vi "Main.vi"() -> ()   [LabVIEW 2018]
panel:
  in  "For Debugging:":bool
  out "State":dbl
  in  "Tab Control":T1(tab)
  out "Mass Flow":dbl(knob) scale=0.0..10.0
  out "Transducer Part":dbl(slide) scale=0.0..10.0
  out "Transducer Source":dbl(slide) scale=0.0..10.0
  out "Thermocouple Part":dbl(slide) scale=0.0..600.0
  out "Thermocouple Source":dbl(slide) scale=0.0..600.0
  in  "Select Default Process":bool
  out "Waveform Graph":waveform(dbl)(graph)
  out "Status Feed":string
  in  "Standard Processes":string(combo)
  out "Valid Process":bool
  in  "ABORT":bool
  in  "Start":bool
  out "Progression":u8(slide) scale=0.0..100.0
  out "DANGER":bool
  in  "Save File(s) Location":path
  in  "Emergency Contact (Carrier)":enum16{"T-Mobile", "AT&T", "Verizon", "Sprint"}(ring)
  in  "Emergency Contact (phone number)":string
  in  "Name of Experiment":string="LabVIEW Error"
  in  "Centigrade / Fahrenheit":bool
  in  "Set Schedules":bool
  in  "Clear Mass Flow Schedule":bool
  in  "Clear Pressure Schedule":bool
  in  "Clear Temp Schedule":bool
  in  "Mass Flow Process Schedule":T2(array[cluster])
  in  "Pressure Process Schedule":T2(array[cluster])
  in  "Temperature Process Schedule":T3(array[cluster])
  in  "Max Rate Temperature 3":dbl
  in  "Min Temperature 3":dbl
  in  "Max Temperature 3":dbl
  in  "Max Rate Temperature 2":dbl
  in  "Min Temperature 2":dbl
  in  "Max Temperature 2":dbl
  in  "Max Rate Temperature":dbl=10.0
  in  "Min Temperature":dbl=25.0
  in  "Max Temperature":dbl=600.0
  out "Input Validated":bool
  out "Initialized":bool
  # "BLUE M SINGLEZONE FURNACE: SKELETON CODE"
  # "Temperature Readings"
  # "Pressure Readings"
  # "Mass Flow Readings"
  # "Temperature Settings"
  # "Mass Flow Settings"
  # "These represent the max allowable settings for the process. It is recommended that temperature limits should be set well within the safety limits of the equipment. Please allow generous safety margins!"
  # "These represent the max allowable settings for the process. It is recommended that temperature limits should be set well within the safety limits of the equipment. Please allow generous safety margins!"
  # "Pressure Settings"
  # "These represent the max allowable settings for the process. It is recommended that temperature limits should be set well within the safety limits of the equipment. Please allow generous safety margins!"
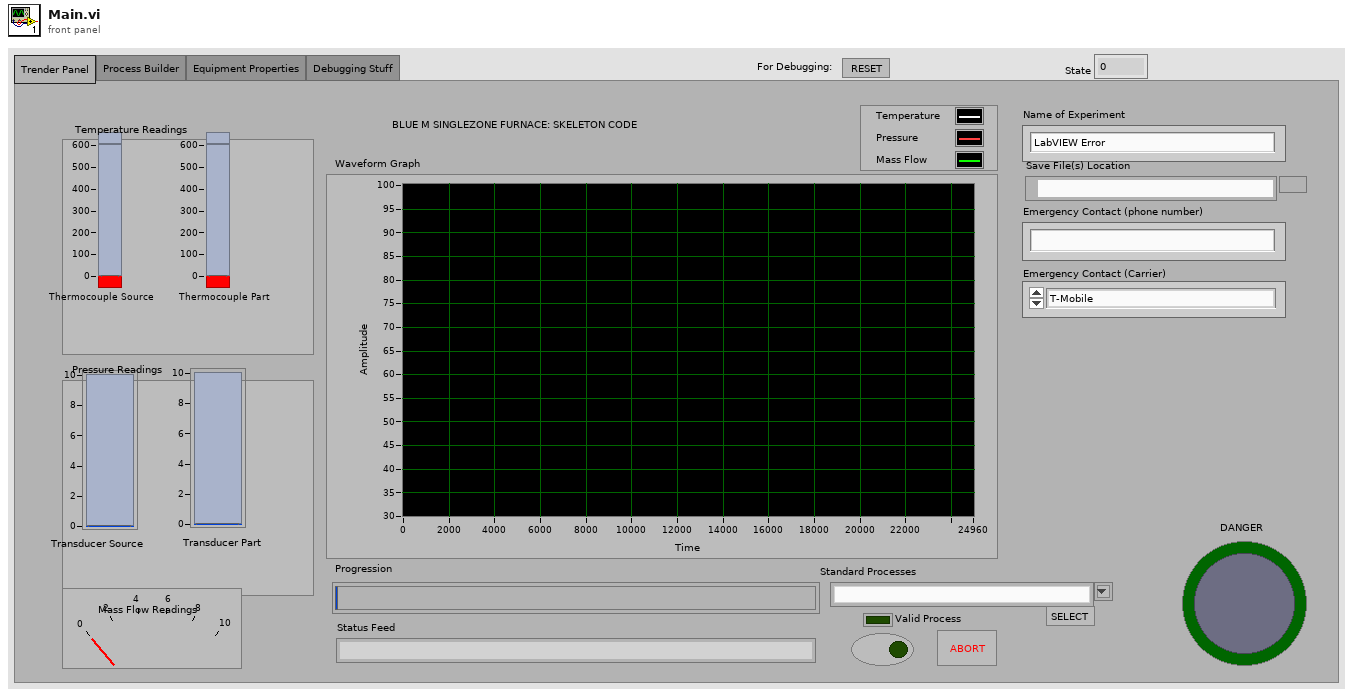
[diagram p1: front panel]
types:
  T1 = enum32{"Trender Panel", "Process Builder", "Equipment Properties", "Debugging Stuff"}
  T2 = cluster{"time (s)":dbl, "setpoint (C) ":dbl, "Resolution (1/min)":dbl}[]
  T3 = cluster{"Duration (min)":dbl, "Rate (C/min) ":dbl, "Resolution (1/min)":dbl}[]
  T4 = cluster{"time (s)":dbl, "setpoint ":dbl, "frequency":dbl}[]
  T5 = cluster{"Duration (min)":dbl, "Rate (C/min) ":dbl, "Frequency (1/min)":dbl}[]
  T6 = cluster{"Max Temperature":dbl, "Min Temperature":dbl, "Max Rate Temperature":dbl}
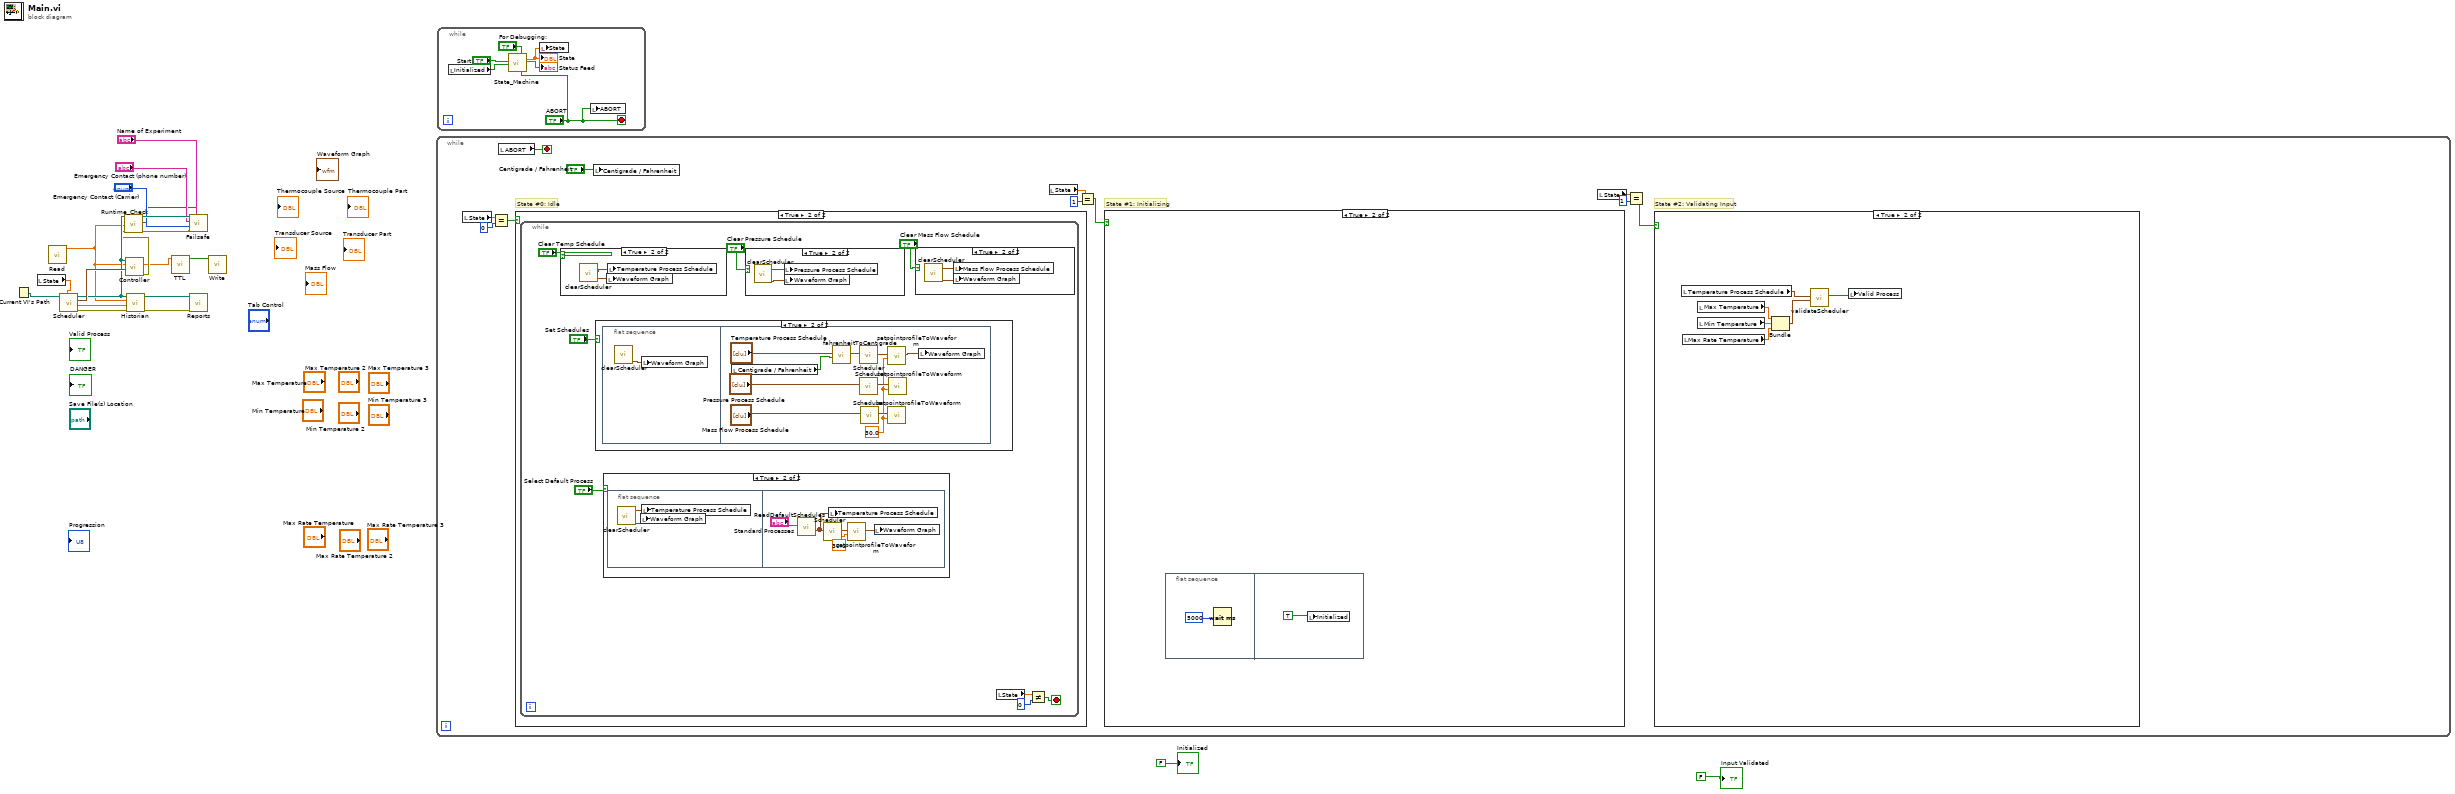
[diagram p0: block diagram]
diagram:
  n1 = Current VI's Path() -> (path=w19:path)
  n2 = local read "State"() -> (w20:dbl)
  n3 = call "Read.vi"() -> ("PV:"=w5:dbl)  [unwired: 11 in]
  n4 = call "Scheduler.vi"("Path In"=w19, "Action"=w20) -> ("Path Out"=w13:path, "Setpoint Profile"=w17:cluster{"Time (s)":dbl, "setpoint (C)":dbl}[], "Sampling Rates"=w18:dbl[], "error out"=w16:errorcluster)  [unwired: 4 in, 1 out]
  n5 = call "Controller.vi"("Path In"=w13, "Signal (Reference)"=w5, "setpoint profile"=w17) -> ("Reaction (Output)"=w7:dbl, "error out"=w10:errorcluster)  [unwired: 5 in, 1 out]
  n6 = call "Runtime_Check.vi"("Path In"=w13, "Signal"=w5, "error in (no error)"=w10) -> ("Path Out"=w12:path, "Danger?"=w1:bool, "error out"=w11:errorcluster)  [unwired: 14 in]
  n7 = call "Historian.vi"("error in (no error)"=w16, "Sampling Rates"=w18, "Sample"=w5, "Path In"=w13) -> ("error out"=w15:errorcluster, "Path Out"=w14:path)  [unwired: 5 in, 1 out]
  n8 = call "TTL.vi"("MV"=w7) -> ("TTL"=w6:bool[])  [unwired: 10 in]
  n9 = call "Failsafe.vi"("Name of Experiment"="Name of Experiment", "Danger?"=w1, "error in"=w11, "Emergency Contact (Carrier)"="Emergency Contact (Carrier)", "Emergency Contact (phone number)"="Emergency Contact (phone number)", "Path In"=w12) -> ()  [unwired: 4 in, 2 out]
  n10 = call "Reports.vi"("error in (no error)"=w15, "Path In"=w14) -> ()  [unwired: 6 in, 4 out]
  n11 = call "Write.vi"("TTL"=w6) -> ()  [unwired: 11 in]
  n12 = while {
    stop <- w31 stop-if-true
    # "State #2: Validating Input"
    # "State #1: Initializing"
    # "State #0: Idle"
    n13 = local read "State"() -> (w29:dbl)
    n14 = Equal?(x=w29, y=0) -> (x = y?=w30:bool)
    n15 = local read "ABORT"() -> (w31:bool)
    n16 = case shown="True" w30 {
      frame False {
      }
      frame True {
        n17 = while {
          stop <- w45 stop-if-true
          n18 = case shown="True" "Clear Temp Schedule" {
            frame False {
            }
            frame True {
              n19 = call "clearScheduler.vi"() -> ("Empty Waveform"=w70:waveform(dbl), "Empty Scheduler"=w71:T4)  [unwired: 8 in, 1 out]
              n20 = local write "Waveform Graph"(w70) -> ()
              n21 = local write "Temperature Process Schedule"(w71) -> ()
            }
          }
          n22 = case shown="True" "Set Schedules" {
            frame False {
            }
            frame True {
              n23 = flat-sequence {
                frame #0 {
                  n24 = call "clearScheduler.vi"() -> ("Empty Waveform"=w59:waveform(dbl))  [unwired: 8 in, 2 out]
                  n25 = local write "Waveform Graph"(w59) -> ()
                }
                frame #1 {
                  w67 = 30.0
                  n26 = local read "Centigrade / Fahrenheit"() -> (w60:bool)
                  n27 = call "fahrenheitToCentigrade.vi"("Convert?"=w60, "Schedule Before"="Temperature Process Schedule") -> ("Schedule After"=w62:T5)  [unwired: 9 in]
                  n28 = call "Scheduler.vi"("Scheduler"=w62) -> ("Setpoint Profile"=w63:cluster{"Time (s)":dbl, "setpoint (C)":dbl}[])  [unwired: 5 in, 4 out]
                  n29 = call "Scheduler.vi"("Scheduler"="Pressure Process Schedule") -> ("Setpoint Profile"=w68:cluster{"Time (s)":dbl, "setpoint (C)":dbl}[])  [unwired: 5 in, 4 out]
                  n30 = call "Scheduler.vi"("Scheduler"="Mass Flow Process Schedule") -> ("Setpoint Profile"=w69:cluster{"Time (s)":dbl, "setpoint (C)":dbl}[])  [unwired: 5 in, 4 out]
                  n31 = call "setpointprofileToWaveform.vi"("Room Temp Offset"=w67, "setpoint profile"=w63) -> ("Waveform"=w64:waveform(dbl))  [unwired: 9 in]
                  n32 = call "setpointprofileToWaveform.vi"("Room Temp Offset"=w67, "setpoint profile"=w69) -> ()  [unwired: 9 in, 1 out]
                  n33 = call "setpointprofileToWaveform.vi"("Room Temp Offset"=w67, "setpoint profile"=w68) -> ()  [unwired: 9 in, 1 out]
                  n34 = local write "Waveform Graph"(w64) -> ()
                }
              }
            }
          }
          n35 = case shown="True" "Select Default Process" {
            frame False {
            }
            frame True {
              n36 = flat-sequence {
                frame #0 {
                  n37 = call "clearScheduler.vi"() -> ("Empty Waveform"=w53:waveform(dbl), "Empty Scheduler"=w52:T4)  [unwired: 8 in, 1 out]
                  n38 = local write "Waveform Graph"(w53) -> ()
                  n39 = local write "Temperature Process Schedule"(w52) -> ()
                }
                frame #1 {
                  n40 = call "ReadDefaultSchedules.vi"("File Name"="Standard Processes") -> ("Scheduler"=w54:T4)  [unwired: 8 in, 2 out]
                  n41 = call "Scheduler.vi"("Scheduler"=w54) -> ("Setpoint Profile"=w58:cluster{"Time (s)":dbl, "setpoint (C)":dbl}[])  [unwired: 5 in, 4 out]
                  n42 = local write "Temperature Process Schedule"(w54) -> ()
                  n43 = call "setpointprofileToWaveform.vi"("Room Temp Offset"=30.0, "setpoint profile"=w58) -> ("Waveform"=w55:waveform(dbl))  [unwired: 9 in]
                  n44 = local write "Waveform Graph"(w55) -> ()
                }
              }
            }
          }
          n45 = case shown="True" "Clear Pressure Schedule" {
            frame False {
            }
            frame True {
              n46 = call "clearScheduler.vi"() -> ("Empty Waveform"=w50:waveform(dbl), "Empty Scheduler"=w51:T4)  [unwired: 8 in, 1 out]
              n47 = local write "Pressure Process Schedule"(w51) -> ()
              n48 = local write "Waveform Graph"(w50) -> ()
            }
          }
          n49 = case shown="True" "Clear Mass Flow Schedule" {
            frame False {
            }
            frame True {
              n50 = call "clearScheduler.vi"() -> ("Empty Waveform"=w48:waveform(dbl), "Empty Scheduler"=w49:T4)  [unwired: 8 in, 1 out]
              n51 = local write "Mass Flow Process Schedule"(w49) -> ()
              n52 = local write "Waveform Graph"(w48) -> ()
            }
          }
          n53 = local read "State"() -> (w46:dbl)
          n54 = Not Equal?(x=w46, y=0) -> (x != y?=w45:bool)
        }
      }
    }
    n55 = local write "Centigrade / Fahrenheit"("Centigrade / Fahrenheit") -> ()
    n56 = local read "State"() -> (w25:dbl)
    n57 = Equal?(x=w25, y=1) -> (x = y?=w26:bool)
    n58 = case shown="True" w26 {
      frame False {
      }
      frame True {
        n59 = flat-sequence {
          frame #0 {
            n60 = Wait (ms)(milliseconds to wait=5000) -> ()  [unwired: 1 out]
          }
          frame #1 {
            n61 = local write "Initialized"(TRUE) -> ()
          }
        }
      }
    }
    n62 = local read "State"() -> (w22:dbl)
    n63 = Equal?(x=w22, y=1) -> (x = y?=w23:bool)
    n64 = case shown="True" w23 {
      frame False {
      }
      frame True {
        n65 = local read "Temperature Process Schedule"() -> (w34:T3)
        n66 = local read "Max Rate Temperature"() -> (w35:dbl)
        n67 = local read "Max Temperature"() -> (w37:dbl)
        n68 = local read "Min Temperature"() -> (w36:dbl)
        n69 = Bundle("Max Temperature"=w37, "Min Temperature"=w36, "Max Rate Temperature"=w35) -> (w33:T6)  [unwired: 1 in]
        n70 = call "validateScheduler.vi"("Constraints"=w33, "Schedule"=w34) -> ("Valid Input"=w32:bool)  [unwired: 8 in, 1 out]
        n71 = local write "Valid Process"(w32) -> ()
      }
    }
  }
  n72 = while {
    stop <- "ABORT" stop-if-true
    n73 = local read "Initialized"() -> (w72:bool)
    n74 = call "State_Machine.vi"("Start Process"="Start", "Initialized"=w72, "Reset"="For Debugging:", "Powering Down"="ABORT") -> ("State"=w77:dbl, "State String"=→"Status Feed":string)  [unwired: 12 in, 2 out]
    "State" <- w77
    n75 = local write "State"(w77) -> ()
    n76 = local write "ABORT"("ABORT") -> ()
  }
  "Initialized" <- FALSE
  "Input Validated" <- FALSE
